vi "pco.camera_Avg_Example.vi"() -> ()   [LabVIEW 2019]
uses:
  pco.camera/Camera.lvclass
  <vilib>/picture/picture.llb/Draw 8-Bit Pixmap.vi
  <vilib>/picture/picture.llb/Draw True-Color Pixmap.vi
panel:
  out "colormap(U8)":u32[](array[numeric])
  out "Image(U16)":u16[][](graph)
  in  "Zoom [%]":i32(c297)=26
  out "Image":picture
  out "rawImage":u16[][](array[numeric])
  in  "data_format":T1(ring)=enum."Mono16"
  out "Recorded Images":u32
  in  "Quit":bool
  in  "roiY1":u64=2 min=2 max=2160 step=1
  in  "roiX1":u64=2 min=2 max=2560 step=1
  in  "roiY0":u64=1 min=1 max=2159 step=1
  in  "roiX0":u64=1 min=1 max=2559 step=1
  out "Image Height":u64
  out "Image Width":u64
  in  "dwImgCount":u32=10 caption="Required Number of Images" max=4023
  out "Error":errorcluster {"code" format="%x"}
  # "This example shows how to continously compute and show an averaged image.\nHere the camera class is operated in sequence mode and the required number of images also defines the number of images that will be averaged\nIt is a good starting point for writing own applications.\nBut it will not be fail save, i.e. doesnt react on errors, just handles them forward to the end\n\nUsage:\nSelect your required image count you want to average over before you start the program.\nOnce started, the camera class will be initialized and image record will start automatically.\nInside the acquisition loop the program will record the image sequence.\nThen it calculates the average image and shows it.\nBy using the ROI parameters you can crop the image to select certain regions\n\nBy clicking Quit Application the record will stop and will force an exit of the camera class"
  # "pco.labview"
  # "Camera Setup"
  # "Recording Control"
  # "Parameters for image readout"
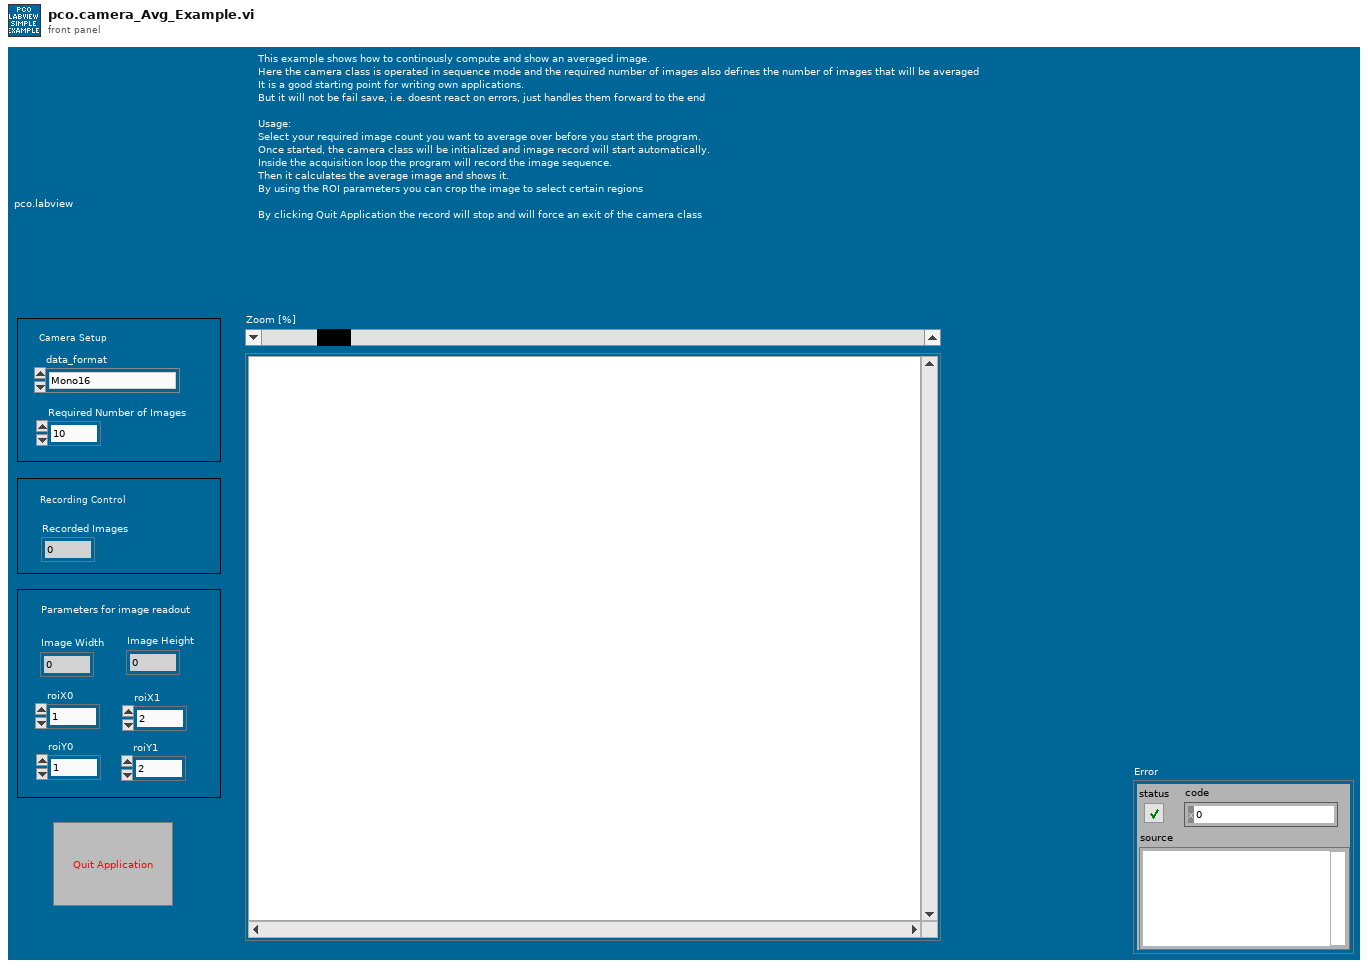
[diagram p1: front panel]
types:
  T1 = enum16{"Undefined", "Mono8", "Mono16", "BGRA8", "RGBA8", "BGRA16", "RGBA16", "CompressedMono8"}
  T2 = enum8{"Enabled", "Disabled", "Disabled and Grayed Out"}
  T3 = enum16{"sequence", "sequence non blocking", "ring buffer", "fifo", "sequence_dpcore", "sequence_non_blocking_dpcore", "ring_buffer_dpcore", "fifo_dpcore", "tif", "multitif", "pcoraw", "b16", "dicom", "multidicom"}
  T4 = typedef "Camera.lvclass/binning.ctl" = cluster{"vert":u16, "horz":u16}
  T5 = cluster{"exposure_time_s":dbl, "delay_time_s":dbl, "roi":cluster{"x0":u64, "y0":u64, "x1":u64, "y1":u64}, "timestamp_mode":u16, "pixelrate":u32, "trigger_mode":u16, "acquire_mode":u16, "metadata_mode":u16, "noisefilter_mode":u16, "binning":T4}
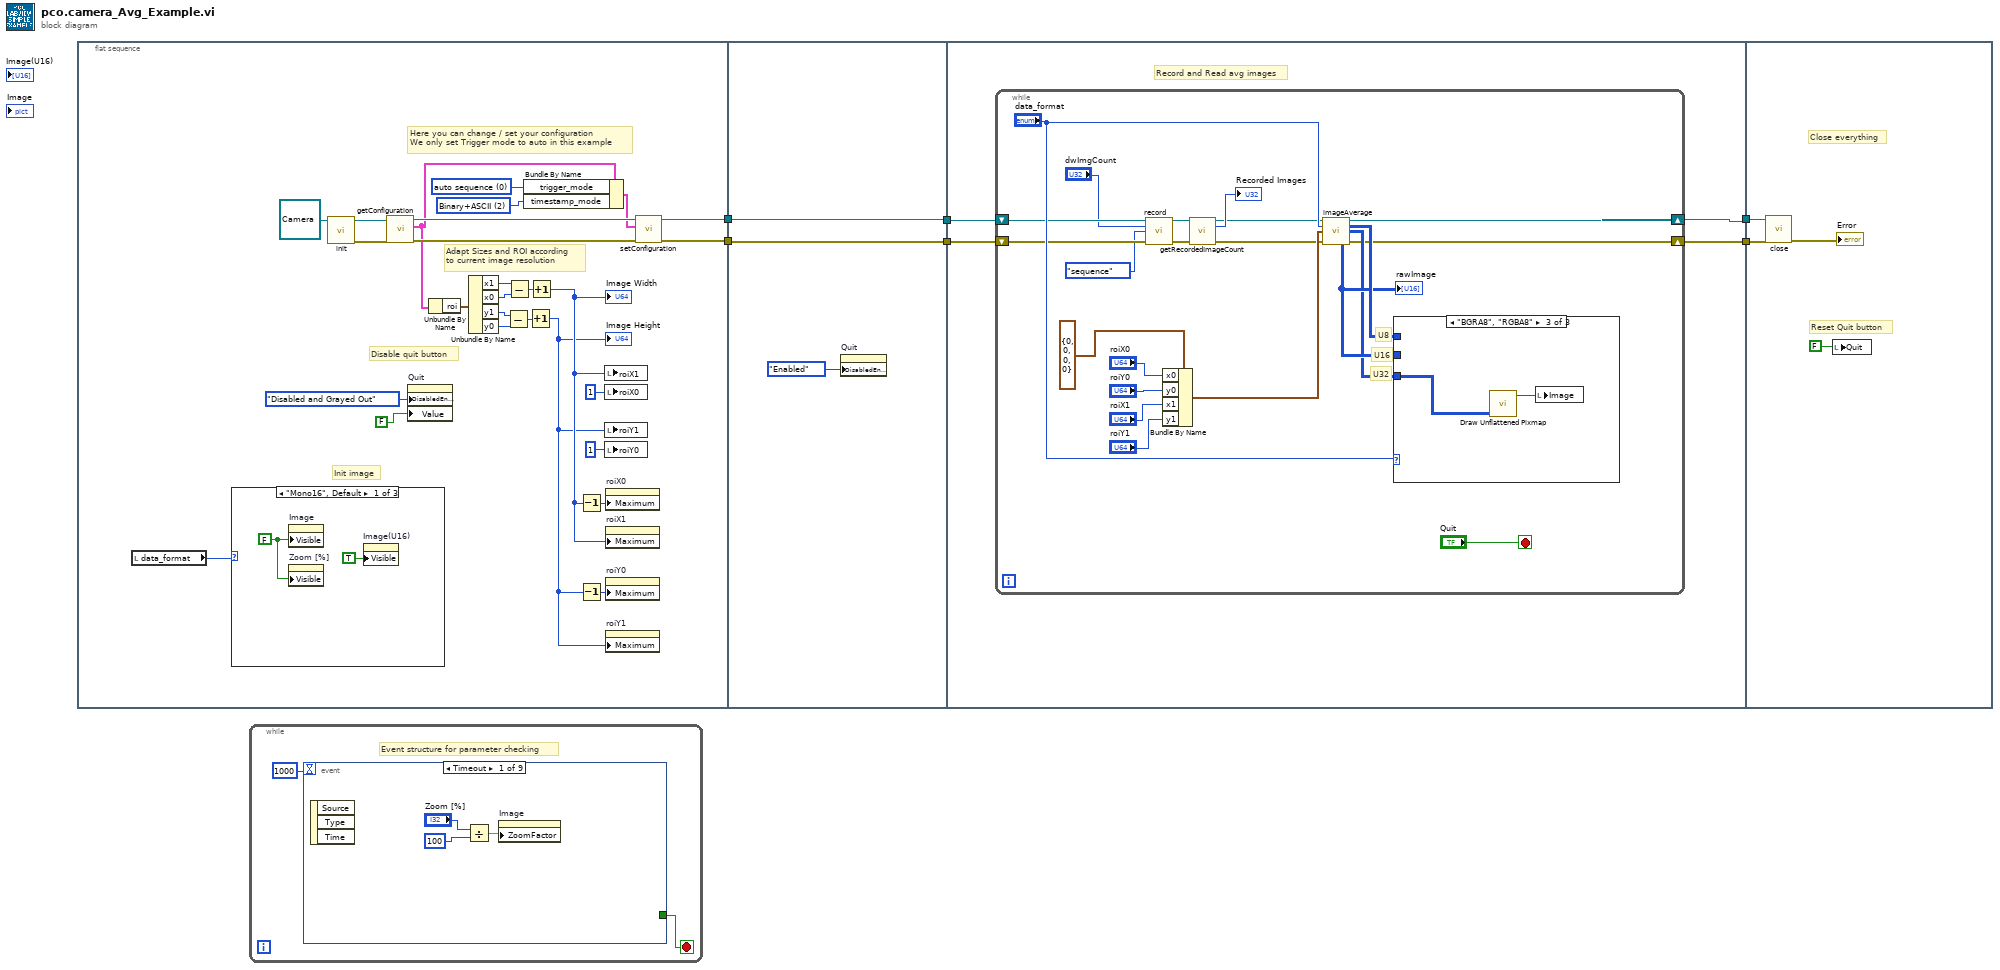
[diagram p0: block diagram]
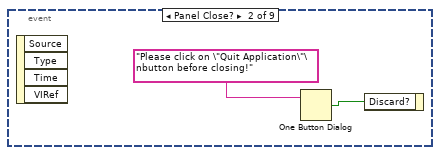
[diagram p2: hidden frame]
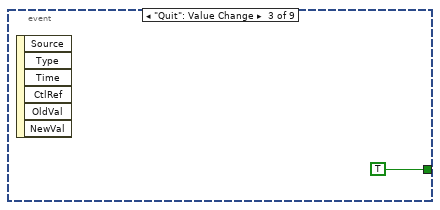
[diagram p3: hidden frame]
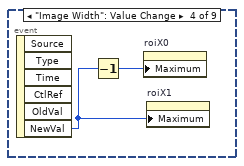
[diagram p4: hidden frame]
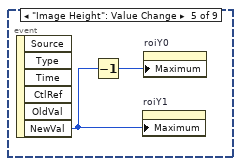
[diagram p5: hidden frame]
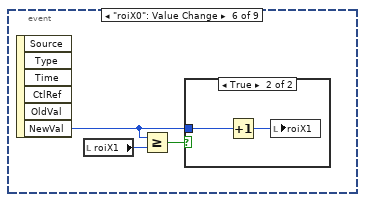
[diagram p6: hidden frame]
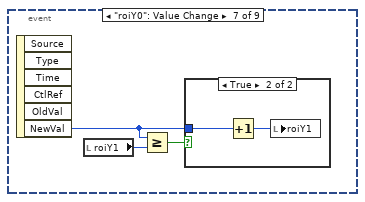
[diagram p8: hidden frame]
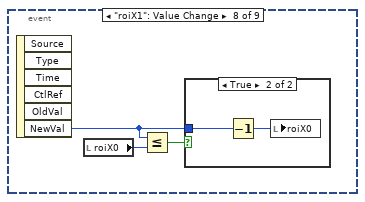
[diagram p10: hidden frame]
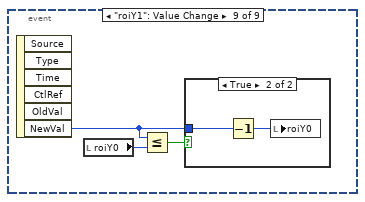
[diagram p12: hidden frame]
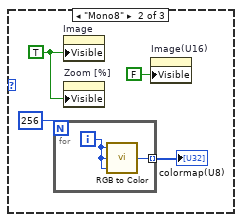
[diagram p14: hidden frame]
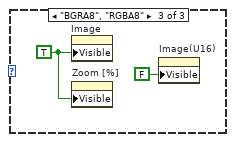
[diagram p15: hidden frame]
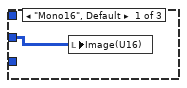
[diagram p16: hidden frame]
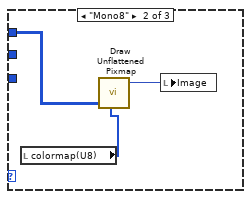
[diagram p17: hidden frame]
diagram:
  n1 = flat-sequence {
    tunnel: [w8] -> w6
    tunnel: [w7] -> w5
    tunnel: w6 -> [w45]
    tunnel: w5 -> [w44]
    tunnel: [w45] -> w4
    tunnel: [w44] -> w3
    tunnel: [w50] -> w2
    tunnel: [w49] -> w1
    tunnel: w3 -> [w48]
    tunnel: w4 -> [w47]
    tunnel: w2 -> [w80]
    tunnel: w1 -> [w79]
    frame #0 {
      w12 = u16 2 items=["OFF", "Binary", "Binary+ASCII", "ASCII"] ("TimestampMode")
      w30 = u16 0 items=["auto sequence"=0, "software trigger"=1, "external exposure start & software trigger"=2, "external exposure control"=3, "external synchronized"=4, "fast external exposure control"=5, "external CDS control"=6, "slow external exposure control"=7, "external synchronized HDSDI"=258] ("TriggerMode")
      # "Init image"
      # "Adapt Sizes and ROI according\nto current image resolution"
      # "Disable quit button"
      # "Here you can change / set your configuration\nWe only set Trigger mode to auto in this example"
      n2 = local read "data_format"() -> (w9:T1)
      n3 = case shown="\"Mono16\", Default" w9 {
        frame "Mono16", Default {
          w34 = FALSE ("Visible")
          n4 = property on="Image" class="Pict"("Visible"=w34) -> ()  [unwired: 2 in, 2 out]
          n5 = property on="Zoom [%]" class="Scroll (strict)"("Visible"=w34) -> ()  [unwired: 2 in, 2 out]
          n6 = property on="Image(U16)" class="IntGraph (strict)"("Visible"=TRUE) -> ()  [unwired: 2 in, 2 out]
        }
        frame "Mono8" {
          w38 = TRUE ("Visible")
          n7 = for {
            N: 256 -> [_]
            tunnel: [w40] -> w37 mode=indexing
            i -> [w41]
            n8 = call <vilib>:"RGB to Color.vi"("B"=w41, "G"=w41, "R"=w41) -> ("Color"=w40:u32)
          }
          "colormap(U8)" <- w37
          n9 = property on="Image" class="Pict"("Visible"=w38) -> ()  [unwired: 2 in, 2 out]
          n10 = property on="Zoom [%]" class="Scroll (strict)"("Visible"=w38) -> ()  [unwired: 2 in, 2 out]
          n11 = property on="Image(U16)" class="IntGraph (strict)"("Visible"=FALSE) -> ()  [unwired: 2 in, 2 out]
        }
        frame "BGRA8", "RGBA8" {
          w42 = TRUE ("Visible")
          n12 = property on="Image" class="Pict"("Visible"=w42) -> ()  [unwired: 2 in, 2 out]
          n13 = property on="Zoom [%]" class="Scroll (strict)"("Visible"=w42) -> ()  [unwired: 2 in, 2 out]
          n14 = property on="Image(U16)" class="IntGraph (strict)"("Visible"=FALSE) -> ()  [unwired: 2 in, 2 out]
        }
      }
      n15 = call-dynamic "init.vi"("Camera in"=refnum<class "Camera.lvclass"> refnum ("PCOCamera in")) -> ("Camera out"=w32:refnum<class "Camera.lvclass">, "error out"=w31:errorcluster)  [unwired: 8 in]
      n16 = call-dynamic "getConfiguration.vi"("error in (no error)"=w31, "Camera in"=w32) -> ("error out"=w28:errorcluster, "configuration"=w22:T5, "Camera out"=w29:refnum<class "Camera.lvclass">)  [unwired: 7 in]
      n17 = property on="Quit" class="Bool (strict)"("DisabledEnum"=T2."Disabled and Grayed Out" ("Disabled"), "Value"=FALSE ("Stop")) -> ()  [unwired: 2 in, 2 out]
      n18 = Unbundle By Name(w22) -> ("roi"=w21:cluster{"x0":u64, "y0":u64, "x1":u64, "y1":u64})
      n19 = Unbundle By Name(w21) -> ("x1"=w19:u64, "x0"=w20:u64, "y1"=w17:u64, "y0"=w18:u64)
      n20 = Subtract(x=w17, y=w18) -> (x-y=w15:u64)
      n21 = Subtract(x=w19, y=w20) -> (x-y=w16:u64)
      n22 = Bundle By Name(cluster=w22, "trigger_mode"=w30, "timestamp_mode"=w12) -> (w27:T5)
      n23 = Increment(x=w15) -> (x+1=w13:u64)
      "Image Height" <- w13
      n24 = Increment(x=w16) -> (x+1=w14:u64)
      "Image Width" <- w14
      n25 = Decrement(x=w14) -> (x-1=w24:u64)
      n26 = Decrement(x=w13) -> (x-1=w23:u64)
      n27 = local write "roiX1"(w14) -> ()
      n28 = local write "roiX0"(u64 1 ("roiY0")) -> ()
      n29 = local write "roiY1"(w13) -> ()
      n30 = local write "roiY0"(u64 1 ("roiY0")) -> ()
      n31 = property on="roiX0" class="DigNum (strict)"("Maximum"=w24) -> ()  [unwired: 2 in, 2 out]
      n32 = property on="roiX1" class="DigNum (strict)"("Maximum"=w14) -> ()  [unwired: 2 in, 2 out]
      n33 = property on="roiY0" class="DigNum (strict)"("Maximum"=w23) -> ()  [unwired: 2 in, 2 out]
      n34 = property on="roiY1" class="DigNum (strict)"("Maximum"=w13) -> ()  [unwired: 2 in, 2 out]
      n35 = call-dynamic "setConfiguration.vi"("error in (no error)"=w28, "configuration"=w27, "Camera in"=w29) -> ("error out"=w7:errorcluster, "Camera out"=w8:refnum<class "Camera.lvclass">)  [unwired: 7 in]
    }
    frame #1 {
      n36 = property on="Quit" class="Bool (strict)"("DisabledEnum"=T2."Enabled" ("Disabled")) -> ()  [unwired: 2 in, 2 out]
    }
    frame #2 {
      # "Record and Read avg images"
      n37 = while {
        shift-right: [w61] -> w50
        shift-left: w47 -> [w60]
        shift-right: [w51] -> w49
        shift-left: w48 -> [w59]
        stop <- "Quit" stop-if-true
        # "U32"
        # "U16"
        # "U8"
        n38 = call-dynamic "record.vi"("Camera in"=w60, "num_images"="dwImgCount", "record_mode"=T3."sequence", "error in (no error)"=w59) -> ("Camera out"=w57:refnum<class "Camera.lvclass">, "error out"=w56:errorcluster)  [unwired: 10 in]
        n39 = Bundle By Name(cluster=cluster{"x0":u64, "y0":u64, "x1":u64, "y1":u64} {"x0"=0, "y0"=0, "x1"=0, "y1"=0} ("roi"), "x0"="roiX0", "y0"="roiY0", "x1"="roiX1", "y1"="roiY1") -> (w68:cluster{"x0":u64, "y0":u64, "x1":u64, "y1":u64})
        n40 = call-dynamic "getRecordedImageCount.vi"("Camera in"=w57, "error in (no error)"=w56) -> ("Camera out"=w54:refnum<class "Camera.lvclass">, "recorded_image_count"=→"Recorded Images":u32, "error out"=w53:errorcluster)  [unwired: 11 in]
        n41 = call-dynamic "imageAverage.vi"("Camera in"=w54, "data_format"="data_format", "roi"=w68, "error in (no error)"=w53) -> ("Camera out"=w61:refnum<class "Camera.lvclass">, "image (U8)"=w66:u8[][], "image (U32)"=w64:u32[][], "raw_image (U16)"=w65:u16[][], "error out"=w51:errorcluster)  [unwired: 6 in, 1 out]
        "rawImage" <- w65
        n42 = case shown="\"BGRA8\", \"RGBA8\"" "data_format" {
          tunnel: w64 -> [_ _ w78]
          tunnel: w66 -> [_ w76 _]
          tunnel: w65 -> [w73 _ _]
          frame "Mono16", Default {
            n43 = local write "Image(U16)"(w73) -> ()
          }
          frame "Mono8" {
            n44 = local read "colormap(U8)"() -> (w74:u32[])
            n45 = call-poly <vilib>:"Draw Unflattened Pixmap.vi"("data"=w76, "color table"=w74) -> ("new picture"=w75:picture)  [unwired: 7 in]
            n46 = local write "Image"(w75) -> ()
          }
          frame "BGRA8", "RGBA8" {
            n47 = call-poly <vilib>:"Draw Unflattened Pixmap.vi"("data (RGB format)"=w78) -> ("new picture"=w77:picture)  [unwired: 8 in]
            n48 = local write "Image"(w77) -> ()
          }
        }
      }
    }
    frame #3 {
      # "Reset Quit button"
      # "Close everything"
      n49 = call-dynamic "close.vi"("error in (no error)"=w79, "Camera in"=w80) -> ("error out"=→"Error":errorcluster)  [unwired: 9 in]
      n50 = local write "Quit"(FALSE ("Stop")) -> ()
    }
  }
  n51 = while {
    stop <- w83 stop-if-true
    # "Event structure for parameter checking"
    n52 = event shown="[0] Timeout" {
      selector: _ -> [_ _ _ _ _ _ _ _ _]
      dyn-events: _ -> [_ _ _ _ _ _ _ _ _]
      timeout: 1000 -> [_ _ _ _ _ _ _ _ _]
      tunnel: [_ _ TRUE _ _ _ _ _ _] -> w83
      event Timeout {
        n53 = event-data() -> ()  [unwired: 1 in, 3 out]
        n54 = Divide(x="Zoom [%]", y=100 ("Zoom [%]")) -> (x/y=w86:dbl)
        n55 = property on="Image" class="Pict"("ZoomFactor"=w86) -> ()  [unwired: 2 in, 2 out]
      }
      event Panel Close? {
        n56 = event-data() -> ()  [unwired: 1 in, 4 out]
        n57 = One Button Dialog(message="Please click on \"Quit Application\"\nbutton before closing!") -> (true=w88:bool)  [unwired: 1 in]
        n58 = event-data("Discard?"=w88) -> ()  [unwired: 1 in, 1 out]
      }
      event "Quit": Value Change {
        n59 = event-data() -> ()  [unwired: 1 in, 6 out]
      }
      event "Image Width": Value Change {
        n60 = event-data() -> ("NewVal"=w91:u64)  [unwired: 1 in, 5 out]
        n61 = Decrement(x=w91) -> (x-1=w92:u64)
        n62 = property on="roiX0" class="DigNum (strict)"("Maximum"=w92) -> ()  [unwired: 2 in, 2 out]
        n63 = property on="roiX1" class="DigNum (strict)"("Maximum"=w91) -> ()  [unwired: 2 in, 2 out]
      }
      event "Image Height": Value Change {
        n64 = event-data() -> ("NewVal"=w93:u64)  [unwired: 1 in, 5 out]
        n65 = Decrement(x=w93) -> (x-1=w94:u64)
        n66 = property on="roiY1" class="DigNum (strict)"("Maximum"=w93) -> ()  [unwired: 2 in, 2 out]
        n67 = property on="roiY0" class="DigNum (strict)"("Maximum"=w94) -> ()  [unwired: 2 in, 2 out]
      }
      event "roiX0": Value Change {
        n68 = event-data() -> ("NewVal"=w95:u64)  [unwired: 1 in, 5 out]
        n69 = local read "roiX1"() -> (w97:u64)
        n70 = Greater Or Equal?(x=w95, y=w97) -> (x >= y?=w96:bool)
        n71 = case shown="True" w96 {
          tunnel: w95 -> [_ w99]
          frame False {
          }
          frame True {
            n72 = Increment(x=w99) -> (x+1=w98:u64)
            n73 = local write "roiX1"(w98) -> ()
          }
        }
      }
      event "roiY0": Value Change {
        n74 = event-data() -> ("NewVal"=w100:u64)  [unwired: 1 in, 5 out]
        n75 = local read "roiY1"() -> (w102:u64)
        n76 = Greater Or Equal?(x=w100, y=w102) -> (x >= y?=w101:bool)
        n77 = case shown="True" w101 {
          tunnel: w100 -> [_ w104]
          frame False {
          }
          frame True {
            n78 = Increment(x=w104) -> (x+1=w103:u64)
            n79 = local write "roiY1"(w103) -> ()
          }
        }
      }
      event "roiX1": Value Change {
        n80 = event-data() -> ("NewVal"=w105:u64)  [unwired: 1 in, 5 out]
        n81 = local read "roiX0"() -> (w107:u64)
        n82 = Less Or Equal?(x=w105, y=w107) -> (x <= y?=w106:bool)
        n83 = case shown="True" w106 {
          tunnel: w105 -> [_ w109]
          frame False {
          }
          frame True {
            n84 = Decrement(x=w109) -> (x-1=w108:u64)
            n85 = local write "roiX0"(w108) -> ()
          }
        }
      }
      event "roiY1": Value Change {
        n86 = event-data() -> ("NewVal"=w110:u64)  [unwired: 1 in, 5 out]
        n87 = local read "roiY0"() -> (w112:u64)
        n88 = Less Or Equal?(x=w110, y=w112) -> (x <= y?=w111:bool)
        n89 = case shown="True" w111 {
          tunnel: w110 -> [_ w114]
          frame False {
          }
          frame True {
            n90 = Decrement(x=w114) -> (x-1=w113:u64)
            n91 = local write "roiY0"(w113) -> ()
          }
        }
      }
    }
  }
